vi "Modify_Indicies_of_Jumps_101_Case-1.vi"(3 "[IN] Current Index":i32, 4 "[IN] Subtracks":T1(array[cluster]), 5 "[IN] Indicies of sub\ntracks for transforma\ntion (resolving)":i32[](array[numeric])) -> (1 "[OUT] Indicies of Jumps":i32[](array[numeric]))   [LabVIEW 2013]
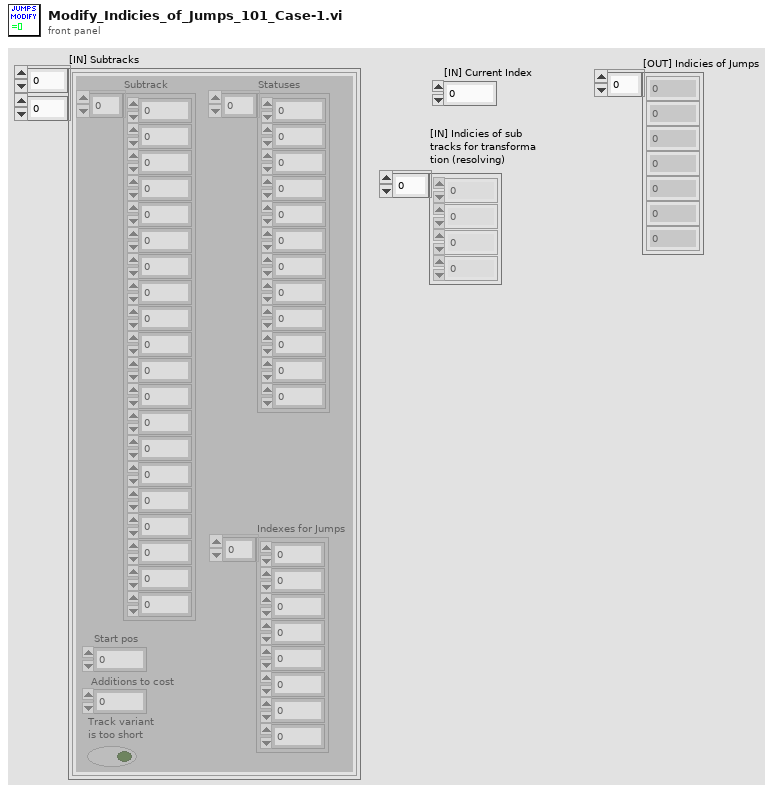
[diagram p1: front panel]
types:
  T1 = cluster{"Subtrack":dbl[], "Statuses":i16[], "Start pos":i32, "Additions to cost":i32, "Track variant \nis too short":bool, "Indexes for Jumps":i32[]}[][]
  T2 = cluster{"Subtrack":dbl[], "Statuses":i16[], "Start pos":i32, "Additions to cost":i32, "Track variant \nis too short":bool, "Indexes for Jumps":i32[]}
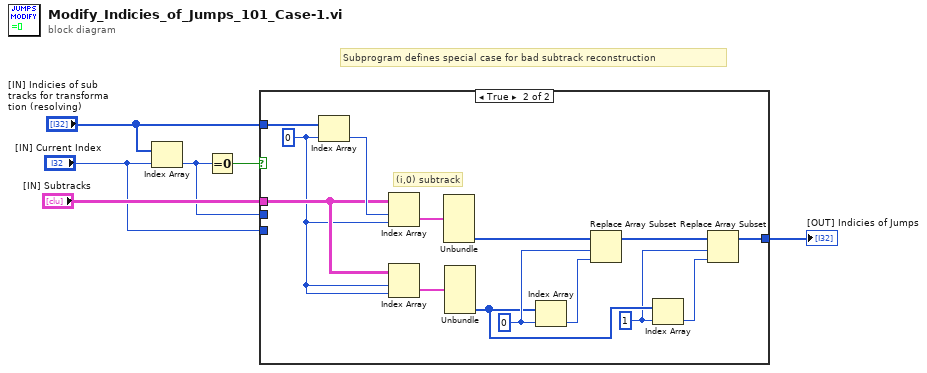
[diagram p0: block diagram]
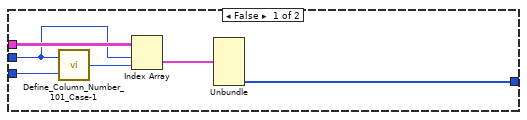
[diagram p2: hidden frame]
diagram:
  # "Subprogram defines special case for bad subtrack reconstruction"
  n1 = Index Array(array="[IN] Indicies of sub\ntracks for transforma\ntion (resolving)", index="[IN] Current Index") -> (element=w2:i32)
  n2 = Equal To 0?(x=w2) -> (x = 0?=w6:bool)
  n3 = case shown="True" w6 {
    tunnel: "[IN] Indicies of sub\ntracks for transforma\ntion (resolving)" -> [_ w26]
    tunnel: "[IN] Subtracks" -> [w11 w23]
    tunnel: [w7 w13] -> w1
    tunnel: "[IN] Current Index" -> [w12 _]
    tunnel: w2 -> [w9 _]
    frame False {
      n4 = call "Define_Column_Number_101_Case-1.vi"("[IN] Current index"=w12, "[IN] Index of \nSubtrack Row"=w9) -> ("[OUT] Column for subtrack"=w10:i32)
      n5 = Index Array(array=w11, index (row)=w9, index (col)=w10) -> (element=w8:T2)
      n6 = Unbundle(w8) -> ("Indexes for Jumps"=w7:i32[])  [unwired: 5 out]
    }
    frame True {
      w15 = 1 ("index")
      w19 = 0 ("index")
      w22 = 0
      # "(i,0) subtrack"
      n7 = Index Array(array=w26, index=w22) -> (element=w25:i32)
      n8 = Index Array(array=w23, index (row)=w25, index (col)=w22) -> (element=w24:T2)
      n9 = Index Array(array=w23, index (row)=w22, index (col)=w22) -> (element=w20:T2)
      n10 = Unbundle(w24) -> ("Indexes for Jumps"=w21:i32[])  [unwired: 5 out]
      n11 = Unbundle(w20) -> ("Indexes for Jumps"=w17:i32[])  [unwired: 5 out]
      n12 = Index Array(array=w17, index=w19) -> (element=w18:i32)
      n13 = Replace Array Subset(array=w21, new element=w18, index=w19) -> (w16:i32[])
      n14 = Index Array(array=w17, index=w15) -> (element=w14:i32)
      n15 = Replace Array Subset(array=w16, new element=w14, index=w15) -> (w13:i32[])
    }
  }
  "[OUT] Indicies of Jumps" <- w1
